vi "Request.vi"(8 "error in (no error)":errorcluster, 10 "Input":T1, 11 "UDP Reader in":refnum<class "UDP Reader.lvclass">) -> (0 "error out":errorcluster, 3 "UDP Reader out":refnum<class "UDP Reader.lvclass">)   [LabVIEW 2022 SP3, in "UDP Reader.lvlib" / "UDP Reader.lvclass"]
uses:
  UDP Reader.lvclass
  UDP Input.ctl
  UDP Reader.lvclass/UDP Reader.ctl
  <vilib>/event_ctls.llb/usereventprio.ctl
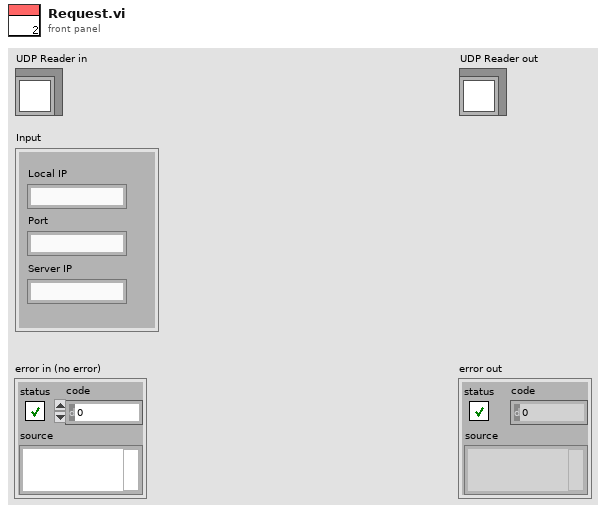
[diagram p1: front panel]
types:
  T1 = typedef "UDP Input.ctl" = cluster{"Local IP":string, "Port":string, "Server IP":string}
  T2 = typedef "usereventprio.ctl" = enum32{"high priority", "normal priority"}
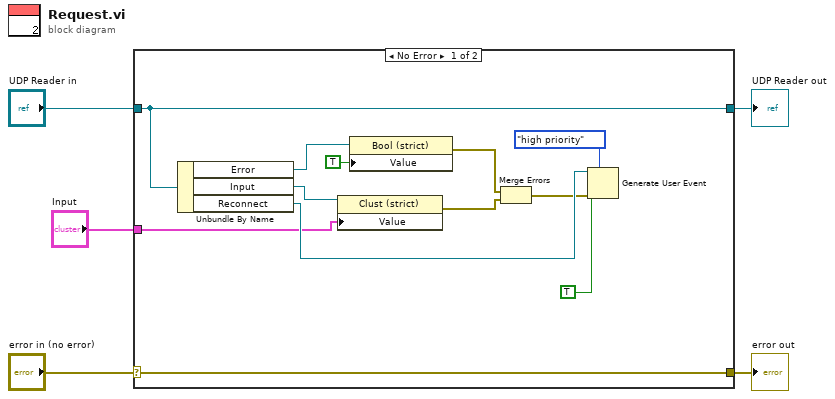
[diagram p0: block diagram]
diagram:
  n1 = case shown="No Error" "error in (no error)" {
    selector: "error in (no error)" -> [w17 w19]
    tunnel: [w17 w19] -> w4
    tunnel: [w16 w18] -> w2
    tunnel: "UDP Reader in" -> [w16 w18]
    tunnel: "Input" -> [w11 _]
    frame No Error {
      n2 = Unbundle By Name(w16) -> ("Error"=w13:refnum<vi>, "Input"=w12:refnum<vi>, "Reconnect"=w14:refnum<user-event>)
      n3 = property class="Clust (strict)"(reference=w12, "Value"=w11) -> (error out=w8:errorcluster)  [unwired: 1 in, 1 out]
      n4 = property class="Bool (strict)"(reference=w13, "Value"=TRUE) -> (error out=w9:errorcluster)  [unwired: 1 in, 1 out]
      n5 = Merge Errors(w9, w8) -> (w7:errorcluster)
      n6 = Generate User Event(priority (normal)=usereventprio."high priority", user event=w14, event data cluster=TRUE ("event data"), error in=w7) -> ()  [unwired: 2 out]
    }
    frame Error {
    }
  }
  "error out" <- w4
  "UDP Reader out" <- w2
